vi "TDT-Get Marker Code.vi"(0 "RPcoX":refnum<k7>, 5 "Last marker num":i32, 11 "error in (no error)":errorcluster) -> (4 "RPcoX thru":refnum<k7>, 6 "Number":i32, 8 "Code":i32, 10 "Delta (ms)":dbl, 14 "new":bool, 15 "error out":errorcluster)   [LabVIEW 2020]
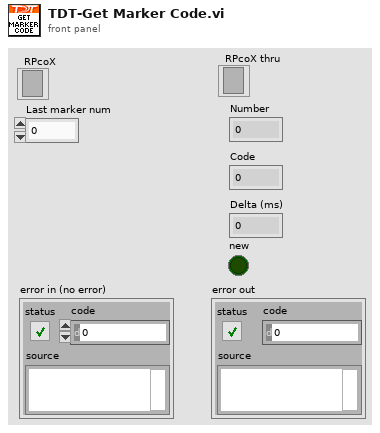
[diagram p1: front panel]
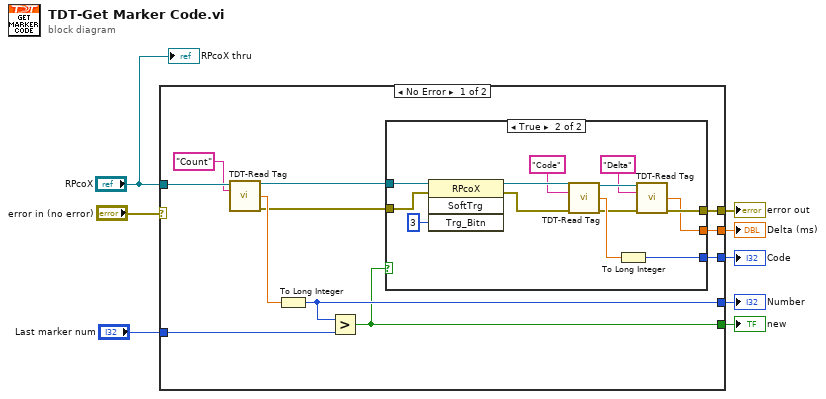
[diagram p0: block diagram]
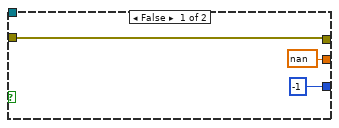
[diagram p2: hidden frame]
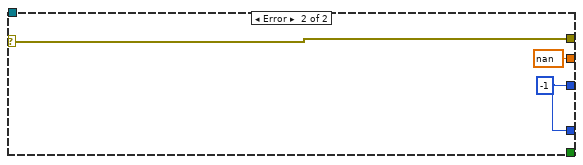
[diagram p3: hidden frame]
diagram:
  n1 = case shown="No Error" "error in (no error)" {
    selector: "error in (no error)" -> [_ w38]
    tunnel: [w11 w38] -> w7
    tunnel: "RPcoX" -> [w19 _]
    tunnel: "Last marker num" -> [w16 _]
    tunnel: [w12 _] -> w5
    tunnel: [w15 w37] -> w4
    tunnel: [w10 w37] -> w2
    tunnel: [w9 nan] -> w3
    frame No Error {
      n2 = call "TDT-Read Tag.vi"("RPcox"=w19, "Name"="Count") -> ("RPcox Out"=w14:refnum<k7>, "GetTagVal"=w17:sgl, "error out"=w13:errorcluster)  [unwired: 11 in]
      n3 = To Long Integer(number=w17) -> (32bit integer=w15:i32)
      n4 = Greater?(x=w15, y=w16) -> (0:w12:bool)
      n5 = case shown="True" w12 {
        tunnel: w14 -> [_ w35]
        tunnel: w13 -> [w22 w34]
        tunnel: [w22 w25] -> w11
        tunnel: [-1 w24] -> w10
        tunnel: [nan w23] -> w9
        frame False {
        }
        frame True {
          n6 = invoke class="RPcoX" method="SoftTrg"(reference=w35, error in=w34, "Trg_Bitn"=3) -> (reference out=w32:refnum<k7>, error out=w31:errorcluster)  [unwired: 1 in, 2 out]
          n7 = call "TDT-Read Tag.vi"("RPcox"=w32, "Name"="Code", "error in"=w31) -> ("RPcox Out"=w28:refnum<k7>, "GetTagVal"=w29:sgl, "error out"=w27:errorcluster)  [unwired: 10 in]
          n8 = To Long Integer(number=w29) -> (32bit integer=w24:i32)
          n9 = call "TDT-Read Tag.vi"("RPcox"=w28, "Name"="Delta", "error in"=w27) -> ("GetTagVal"=w23:sgl, "error out"=w25:errorcluster)  [unwired: 10 in, 1 out]
        }
      }
    }
    frame Error {
      w37 = -1
    }
  }
  "error out" <- w7
  "new" <- w5
  "Number" <- w4
  "Delta (ms)" <- w3
  "Code" <- w2
  "RPcoX thru" <- "RPcoX"
